vi "DROPBEAR_Model_Updating_FEA.vi"(8 "error in (no error)":errorcluster, 11 "DROPBEAR_Model_Updating in":refnum<class "DROPBEAR_Model_Updating.lvclass">) -> (0 "error out":errorcluster, 3 "DROPBEAR_Model_Updating out":refnum<class "DROPBEAR_Model_Updating.lvclass">)   [LabVIEW 2021, in "DROPBEAR_Model_Updating.lvclass"]
uses:
  DROPBEAR_Model_Updating.lvclass
  DROPBEAR_Model_Updating.lvclass/DROPBEAR_Model_Updating.ctl
  Kalman_Filter/Kalman_Filter.lvclass
  FEA_Model/FEA_Model.lvclass
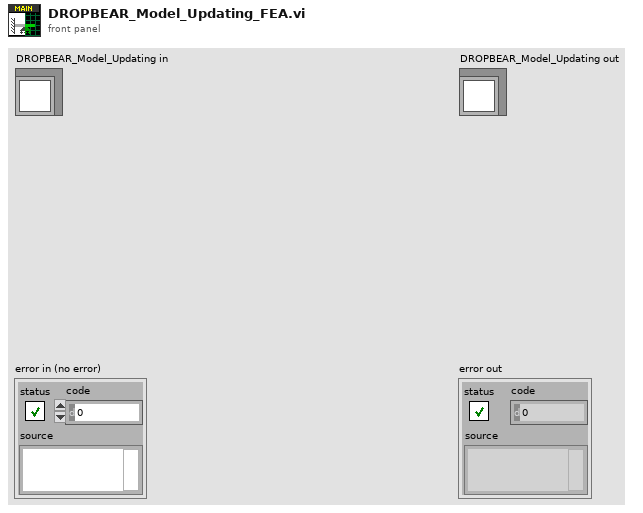
[diagram p1: front panel]
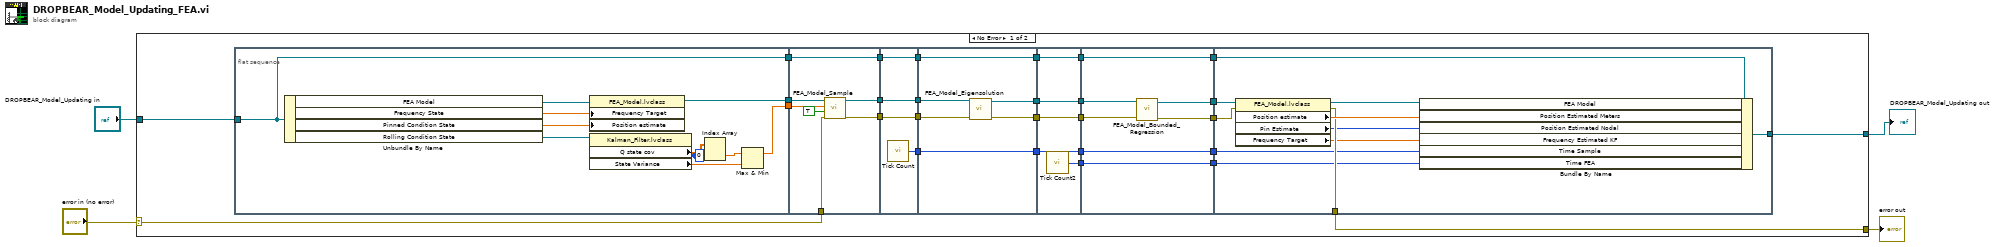
[diagram p0: block diagram]
diagram:
  n1 = case shown="No Error" "error in (no error)" {
    selector: "error in (no error)" -> [w7 w85]
    tunnel: [w6 w85] -> w3
    tunnel: [w8 w84] -> w1
    tunnel: "DROPBEAR_Model_Updating in" -> [w5 w84]
    frame No Error {
      n2 = flat-sequence {
        tunnel: [w41] -> w24
        tunnel: [w34] -> w23
        tunnel: [w33] -> w18
        tunnel: w5 -> [w33]
        tunnel: [w49] -> w32
        tunnel: [w48] -> w31
        tunnel: w24 -> [w47]
        tunnel: w23 -> [w46]
        tunnel: [w45] -> w19
        tunnel: w18 -> [w45]
        tunnel: w7 -> [w44]
        tunnel: w32 -> [w54]
        tunnel: [w54] -> w30
        tunnel: w31 -> [w53]
        tunnel: [w53] -> w29
        tunnel: [w52] -> w20
        tunnel: w19 -> [w52]
        tunnel: [w51] -> w15
        tunnel: w30 -> [w59]
        tunnel: w29 -> [w60]
        tunnel: [w58] -> w28
        tunnel: [w57] -> w26
        tunnel: [w56] -> w21
        tunnel: w20 -> [w56]
        tunnel: [w55] -> w16
        tunnel: w15 -> [w55]
        tunnel: w28 -> [w65]
        tunnel: [w65] -> w27
        tunnel: w26 -> [w64]
        tunnel: [w64] -> w25
        tunnel: [w63] -> w22
        tunnel: w21 -> [w63]
        tunnel: [w62] -> w17
        tunnel: w16 -> [w62]
        tunnel: [w61] -> w14
        tunnel: w27 -> [w71]
        tunnel: w25 -> [w72]
        tunnel: [w70] -> w13
        tunnel: [w69] -> w12
        tunnel: [w68] -> w11
        tunnel: w22 -> [w68]
        tunnel: [w67] -> w10
        tunnel: w17 -> [w67]
        tunnel: [w66] -> w9
        tunnel: w14 -> [w66]
        tunnel: w13 -> [w82]
        tunnel: w12 -> [w80]
        tunnel: w11 -> [w83]
        tunnel: w10 -> [w75]
        tunnel: w9 -> [w76]
        tunnel: [w78] -> w8
        tunnel: [w77] -> w6
        frame #0 {
          w35 = 0 ("index (row)")
          n3 = Unbundle By Name(w33) -> ("FEA Model"=w43:refnum<class "FEA_Model.lvclass">, "Frequency State"=w42:dbl, "Pinned Condition State"=w40:dbl, "Rolling Condition State"=w39:refnum<class "Kalman_Filter.lvclass">)
          n4 = property class="Kalman_Filter.lvclass"(reference=w39) -> ("Q state cov"=w36:dbl[][], "State Variance"=w38:dbl)  [unwired: 1 in, 2 out]
          n5 = property class="FEA_Model.lvclass"(reference=w43, "Frequency Target"=w42, "Position estimate"=w40) -> (reference out=w41:refnum<class "FEA_Model.lvclass">)  [unwired: 1 in, 1 out]
          n6 = Index Array(array=w36, index (row)=w35, index (col)=w35) -> (element=w37:dbl)
          n7 = Max & Min(x=w37, y=w38) -> (max(x,y)=w34:dbl)  [unwired: 1 out]
        }
        frame #1 {
          n8 = call-dynamic "FEA_Model_Sample.vi"("error in (no error)"=w44, "include extremes"=TRUE, "standard_deviation"=w46, "FEA_Model in"=w47) -> ("error out"=w49:errorcluster, "FEA_Model out"=w48:refnum<class "FEA_Model.lvclass">)  [unwired: 6 in]
        }
        frame #2 {
          n9 = call "Tick Count"() -> ("Tick Count(uSec)"=w51:u32)
        }
        frame #3 {
          n10 = call-dynamic "FEA_Model_Eigensolution.vi"("error in (no error)"=w59, "FEA_Model in"=w60) -> ("error out"=w57:errorcluster, "FEA_Model out"=w58:refnum<class "FEA_Model.lvclass">)  [unwired: 8 in]
        }
        frame #4 {
          n11 = call "Tick Count2"() -> ("Tick Count(uSec)"=w61:u32)
        }
        frame #5 {
          n12 = call-dynamic "FEA_Model_Bounded_Regression.vi"("error in (no error)"=w72, "FEA_Model in"=w71) -> ("error out"=w69:errorcluster, "FEA_Model out"=w70:refnum<class "FEA_Model.lvclass">)  [unwired: 8 in]
        }
        frame #6 {
          n13 = property class="FEA_Model.lvclass"(reference=w82, error in=w80) -> (reference out=w81:refnum<class "FEA_Model.lvclass">, error out=w77:errorcluster, "Position estimate"=w79:dbl, "Pin Estimate"=w73:i32, "Frequency Target"=w74:dbl)
          n14 = Bundle By Name(cluster=w83, "FEA Model"=w81, "Position Estimated Meters"=w79, "Position Estimated Nodal"=w73, "Frequency Estimated KF"=w74, "Time Sample"=w75, "Time FEA"=w76) -> (w78:refnum<class "DROPBEAR_Model_Updating.lvclass">)
        }
      }
    }
    frame Error {
    }
  }
  "error out" <- w3
  "DROPBEAR_Model_Updating out" <- w1
